vi "NumberOfPhases.vi"(11 "DeviceSettings":T1 {"Modules"."Grid (0: Normal)" items=["Normal", "Grid Emulation"]; "Modules"."Phase (0: All)" items=["All", "A Phase", "B Phase", "C Phase"]; "Modules"."Mode" items=["One 3-Phase AC", "One AC", "One DC", "Three AC", "Three DC", "One 2-Phase AC and One AC", "One 2-Phase AC and One DC", "Two AC", "One AC and One DC", "Two AC and One DC", "One AC and Two DC", "One DC and One AC", "Two DC"]}) -> (2 "NumberOfPhases":i32, 3 "error out":errorcluster, 5 "Boolean":bool)   [LabVIEW 2018, in "AcPwrPlugins.lvlib" / "NHRGridSim.lvclass"]
uses:
  NHRGridSim.lvclass
  TypeDefs/Device(s)Settings.ctl
  TypeDefs/Modules.ctl
  <vilib>/Utility/error.llb/Error Cluster From Error Code.vi
  <vilib>/ErrorRing/Error Ring.xnode
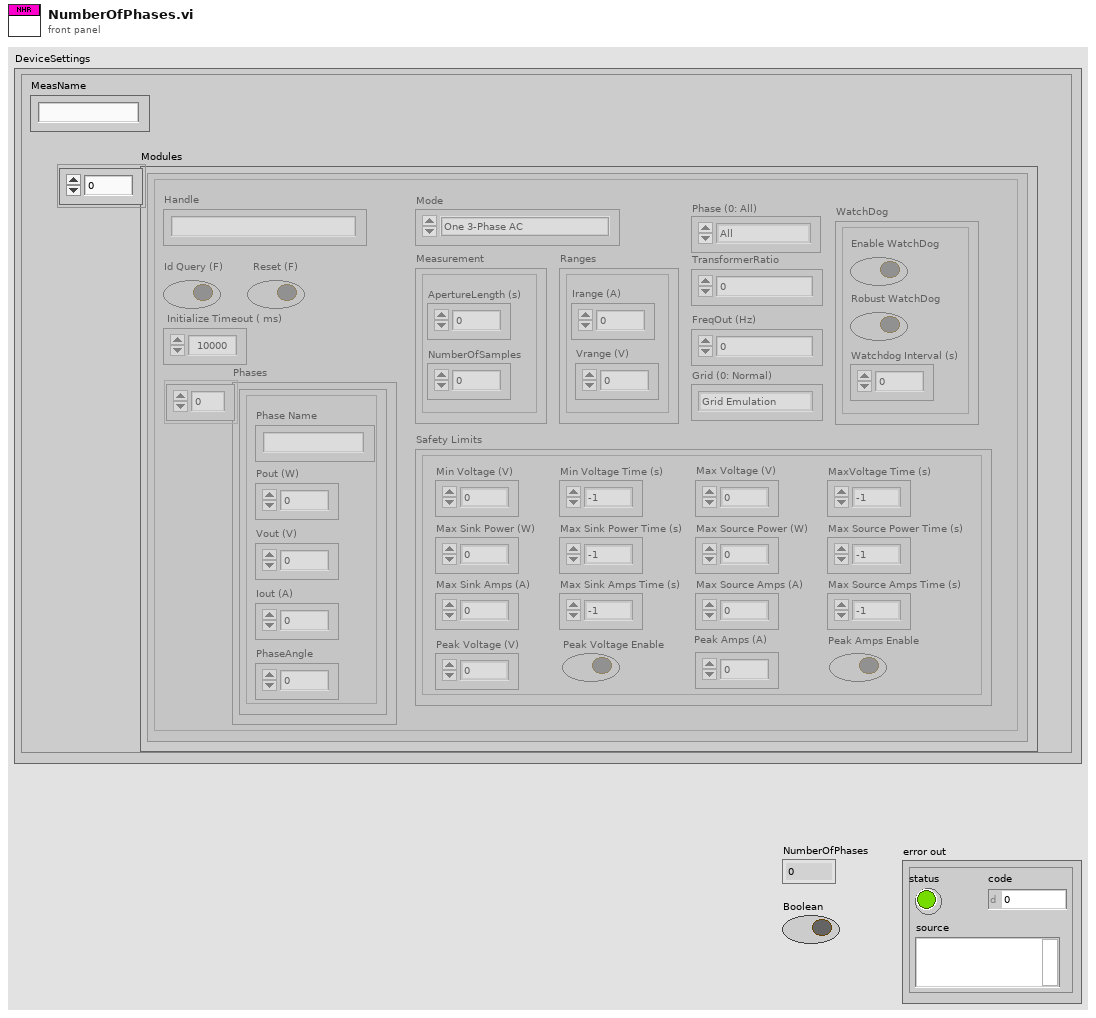
[diagram p1: front panel]
types:
  T1 = typedef "AcPwrPlugins.lvlib/NHRGridSim.lvclass/Device(s)Settings.ctl" = cluster{"MeasName":string, "Modules":T2}
  T2 = typedef "AcPwrPlugins.lvlib/NHRGridSim.lvclass/Modules.ctl" = cluster{"Measurement":cluster{"ApertureLength (s)":dbl, "NumberOfSamples":u32}, "Ranges":cluster{"Irange (A)":dbl, "Vrange (V)":dbl}, "Mode":u8, "TransformerRatio":dbl, "Handle":string, "FreqOut (Hz)":dbl, "Connected":bool, "btnIdQuery":bool, "btnReset":bool, "Initialize Timeout ( ms)":u32, "Phase (0: All)":i32, "Grid (0: Normal)":i32, "WatchDog":cluster{"Enable WatchDog":bool, "Robust WatchDog":bool, "Watchdog Interval (s)":dbl}, "Safety Limits":cluster{"Min Voltage (V)":dbl, "Min Voltage Time (s)":dbl, "Max Voltage (V)":dbl, "MaxVoltage Time (s)":dbl, "Max Source Amps (A)":dbl, "Max Source Amps Time (s)":dbl, "Max Sink Amps (A)":dbl, "Max Sink Amps Time (s)":dbl, "Max Source Power (W)":dbl, "Max Source Power Time (s)":dbl, "Max Sink Power (W)":dbl, "Max Sink Power Time (s)":dbl, "Peak Voltage (V)":dbl, "Peak Voltage Enable":bool, "Peak Amps (A)":dbl, "Peak Amps Enable":bool}, "Phases":cluster{"Pout (W)":dbl, "Iout (A)":dbl, "PhaseAngle":dbl, "Vout (V)":dbl, "Phase Name":string}[]}[]
  T3 = cluster{"Pout (W)":dbl, "Iout (A)":dbl, "PhaseAngle":dbl, "Vout (V)":dbl, "Phase Name":string}[]
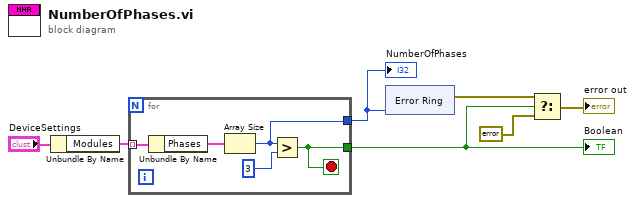
[diagram p0: block diagram]
diagram:
  n1 = Unbundle By Name("DeviceSettings") -> ("Modules"=w1:T2)
  n2 = for {
    tunnel: w1 -> [w10] mode=indexing
    tunnel: [w9] -> w3
    tunnel: [w8] -> w7
    stop <- w9 stop-if-true
    n3 = Unbundle By Name(w10) -> ("Phases"=w12:T3)
    n4 = Array Size(array=w12) -> (size(s)=w8:i32)
    n5 = Greater?(x=w8, y=3) -> (0:w9:bool)
  }
  "Boolean" <- w3
  "NumberOfPhases" <- w7
  n6 = xnode "Error Ring"("parameter 0"=w7) -> ("error out"=w5:errorcluster)
  n7 = Select(t=w5, s=w3, f=errorcluster {"status"=FALSE, "code"=0, "source"=""}) -> (s? t:f=→"error out":errorcluster)
